vi "3-6 Tempature Conversion.vi"() -> ()   [LabVIEW 2015]
panel:
  out "Output Number":dbl
  in  "Input Number":dbl
  in  "Conversion Type":T1(ring)
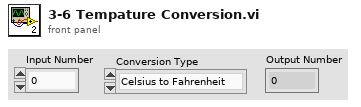
[diagram p1: front panel]
types:
  T1 = enum16{"Celsius to Fahrenheit ", "Fahrenheit  to Celsius", "Celsius to Kelvin", "Fahrenheit to Kelvin"}
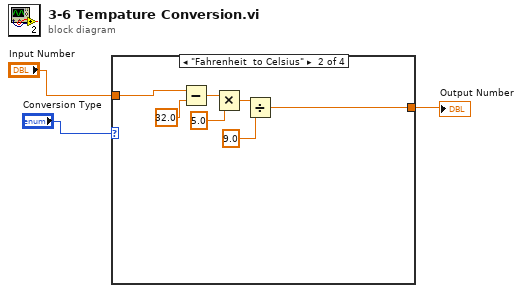
[diagram p0: block diagram]
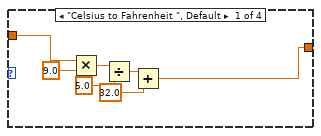
[diagram p2: hidden frame]
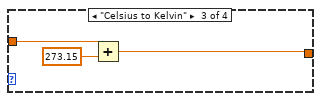
[diagram p3: hidden frame]
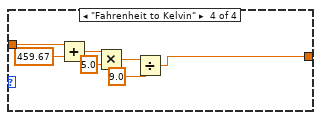
[diagram p4: hidden frame]
diagram:
  n1 = case shown="\"Fahrenheit  to Celsius\"" "Conversion Type" {
    tunnel: "Input Number" -> [w8 w16 w20 w27]
    tunnel: [w7 w11 w18 w21] -> w1
    frame "Celsius to Fahrenheit ", Default {
      n2 = Multiply(x=w8, y=9.0) -> (x*y=w10:dbl)
      n3 = Divide(x=w10, y=5.0) -> (x/y=w9:dbl)
      n4 = Add(x=w9, y=32.0) -> (x+y=w7:dbl)
    }
    frame "Fahrenheit  to Celsius" {
      n5 = Subtract(x=w16, y=32.0) -> (x-y=w15:dbl)
      n6 = Multiply(x=w15, y=5.0) -> (x*y=w14:dbl)
      n7 = Divide(x=w14, y=9.0) -> (x/y=w11:dbl)
    }
    frame "Celsius to Kelvin" {
      n8 = Add(x=w20, y=273.15) -> (x+y=w18:dbl)
    }
    frame "Fahrenheit to Kelvin" {
      n9 = Add(x=w27, y=459.67) -> (x+y=w26:dbl)
      n10 = Multiply(x=w26, y=5.0) -> (x*y=w25:dbl)
      n11 = Divide(x=w25, y=9.0) -> (x/y=w21:dbl)
    }
  }
  "Output Number" <- w1
